vi "Step_ADC_Comparison.vi"(8 "Range(mm)":dbl=10.0, 9 "ADC Voltage":dbl, 10 "Steps":i32) -> (1 "ADC Distance (mm)":dbl, 2 "Moving status":string, 3 "In range":bool)   [LabVIEW 2019]
panel:
  out "Upper Limit":dbl
  out "Lower Limit":dbl
  out "Step Distance(mm)":dbl
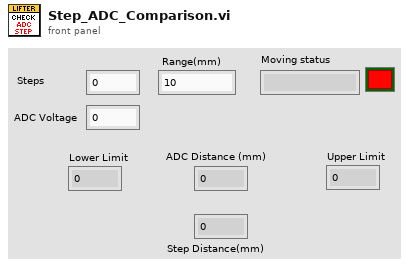
[diagram p1: front panel]
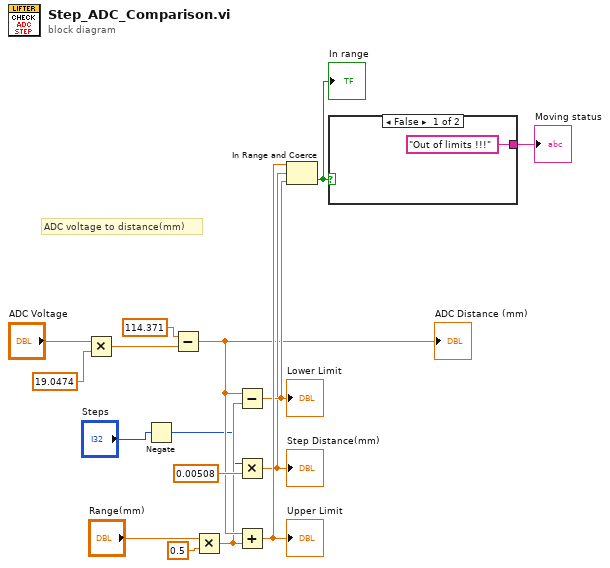
[diagram p0: block diagram]
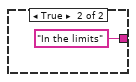
[diagram p2: hidden frame]
diagram:
  # "ADC voltage to distance(mm)"
  n1 = Multiply(x="ADC Voltage", y=19.0474) -> (x*y=w15:dbl)
  n2 = Negate(x="Steps") -> (-x=w1:i32)
  n3 = Subtract(x=114.371, y=w15) -> (x-y=w8:dbl)
  "ADC Distance (mm)" <- w8
  n4 = Multiply(x="Range(mm)", y=0.5) -> (x*y=w5:dbl)
  n5 = Subtract(x=w8, y=w5) -> (x-y=w10:dbl)
  "Lower Limit" <- w10
  n6 = Multiply(x=w1, y=0.00508) -> (x*y=w9:dbl)
  "Step Distance(mm)" <- w9
  n7 = Add(x=w8, y=w5) -> (x+y=w11:dbl)
  "Upper Limit" <- w11
  n8 = In Range and Coerce(upper limit=w11, x=w9, lower limit=w10) -> (In Range?=w7:bool)  [unwired: 1 out]
  "In range" <- w7
  n9 = case shown="False" w7 {
    tunnel: ["Out of limits !!!" "In the limits"] -> w6
    frame False {
    }
    frame True {
    }
  }
  "Moving status" <- w6
